vi "PT 100 R Convert to Temp.vi"(6 "γ":dbl=4.2735e-12 format="%#_6e", 9 "β":dbl=-5.80195e-07 format="%#_6e", 10 "α":dbl=0.00390802 format="%#_6e", 11 "Rt":dbl) -> (3 "t":dbl)   [LabVIEW 2012]
doc: "功能：\n\n计算温度t大于等于0，且小于等于850时的RTD电阻值。"
uses:
  <vilib>/Analysis/polynomials.llb/Polynomial Roots (DBL).vi
  <vilib>/Analysis/NI_AALPro.lvlib
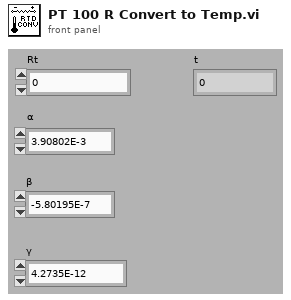
[diagram p1: front panel]
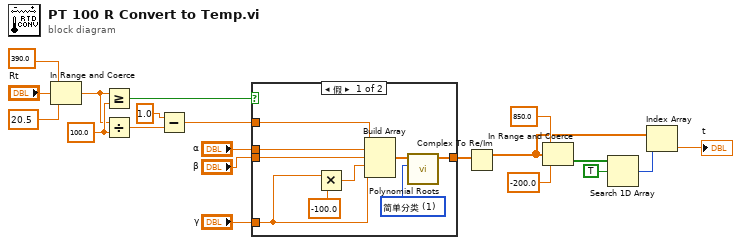
[diagram p0: block diagram]
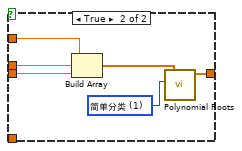
[diagram p2: hidden frame]
diagram:
  w15 = 100.0 ("y")
  n1 = In Range and Coerce(upper limit=390.0 ("上限"), x="Rt", lower limit=20.5 ("下限")) -> (coerced(x)=w3:dbl)  [unwired: 1 out]
  n2 = Greater Or Equal?(x=w3, y=w15) -> (x >= y?=w20:bool)
  n3 = Divide(x=w3, y=w15) -> (x/y=w13:dbl)
  n4 = Subtract(x=1.0, y=w13) -> (x-y=w12:dbl)
  n5 = case shown="假" w20 {
    tunnel: "α" -> [w28 w35]
    tunnel: "β" -> [w27 w34]
    tunnel: "γ" -> [w25 _]
    tunnel: [w22 w30] -> w11
    tunnel: w12 -> [w23 w32]
    frame False {
      w21 = u16 1 items=["常规", "简单分类", "精确", "高级精确"] ("option")
      n6 = Multiply(x=w25, y=-100.0) -> (x*y=w26:dbl)
      n7 = Build Array(w23, w28, w27, w26, w25) -> (w24:dbl[])
      n8 = call-poly <vilib>:"Polynomial Roots.vi"("option"=w21, "P(x)"=w24) -> ("Roots"=w22:cdb[])  [unwired: 8 in, 1 out]
    }
    frame True {
      w31 = u16 1 items=["常规", "简单分类", "精确", "高级精确"] ("option")
      n9 = Build Array(w32, w35, w34) -> (w33:dbl[])
      n10 = call-poly <vilib>:"Polynomial Roots.vi"("option"=w31, "P(x)"=w33) -> ("Roots"=w30:cdb[])  [unwired: 8 in, 1 out]
    }
  }
  n11 = Complex To Re/Im(x + iy=w11) -> (x=w6:dbl[])  [unwired: 1 out]
  n12 = In Range and Coerce(upper limit=850.0 ("t=850"), x=w6, lower limit=-200.0 ("t=-200")) -> (In Range?=w8:bool[])  [unwired: 1 out]
  n13 = Search 1D Array(1D array=w8, element=TRUE ("元素")) -> (index of element=w5:i32)  [unwired: 1 in]
  n14 = Index Array(array=w6, index=w5) -> (element=→"t":dbl)
